vi "Read Input IO Level.vi"(8 "error in (no error)":errorcluster, 11 "CCDCamera in":refnum<class "CCDCamera.lvclass">) -> (0 "error out":errorcluster, 2 "Input Level":bool, 3 "CCDCamera out":refnum<class "CCDCamera.lvclass">)   [LabVIEW 2018, in "CCDCamera.lvclass"]
uses:
  CCDCamera.lvclass
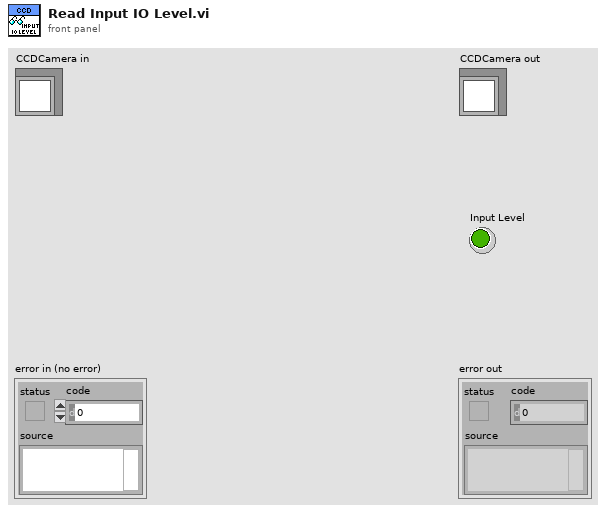
[diagram p1: front panel]
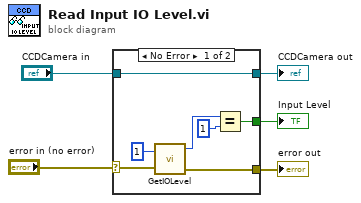
[diagram p0: block diagram]
diagram:
  n1 = case shown="No Error" "error in (no error)" {
    selector: "error in (no error)" -> [w8 w14]
    tunnel: [w7 w14] -> w4
    tunnel: [w12 w13] -> w2
    tunnel: "CCDCamera in" -> [w12 w13]
    tunnel: [w6 _] -> w1
    frame No Error {
      n2 = call <userlib>:"GetIOLevel.vi"("index"=1, "error in (no error)"=w8) -> ("iLevel"=w10:i32, "error out"=w7:errorcluster)  [unwired: 1 out]
      n3 = Equal?(x=w10, y=1) -> (x = y?=w6:bool)
    }
    frame Error {
    }
  }
  "error out" <- w4
  "CCDCamera out" <- w2
  "Input Level" <- w1
